vi "NicmosGlobal.vi"() -> ()   [LabVIEW 2009]
uses:
  Controls/NICMOS.MASKBANKS.ctl
  Controls/NICMOS.FILTERLIST.ctl
  Controls/NICMOS.FILTER.ctl
panel:
  out "BansMasksSquare":T1(array[cluster])
  in  "FilterList":T2
  in  "NI-DAQmx Task":refnum<k21>="NICMOS-DATA-TASK"
  in  "MASKBANKS":T4
  in  "Frame rate":dbl[unit]
  out "t__xx":i32=84
  out "txx__":i32=21
  out "Deglitch":i32=10
  out "Buffer Size":u32=1278
  out "Read Number":i32=138
  in  "Wheel Timeout":i32=90000
  in  "General Timeout":u32=10000
  out "Port Nicmos":refnum<visa-resource-name>="COM104"
  out "Reform Y":i32[](array[numeric])=[1, 1, 9, 9, 9, 9, 100]
  out "Reform X":i32[](array[numeric])=[1, 1, 9, 1, 9, 50, 100]
  out "Max Frequency":dbl[unit][](array[numeric])=[153846.15384615387, 105263.15789473684, 2442.002442002442, 3421.7279726261763, 2385.211687537269, 935.2349777881694, 48.14462645787947] format="%.2f"
  out "Min Frequency":dbl[unit][](array[numeric])=[238.2370458606313, 238.06689679800022, 217.36767742636667, 223.0524730942954, 216.90797679084645, 190.1050330307495, 40.061293779482604] format="%.2f"
  out "Bank Base Time":dbl[unit][](array[numeric])=[6.499999999999999e-06, 9.5e-06, 0.0004095, 0.00029225, 0.00041924999999999997, 0.0010692499999999999, 0.02077075] format="%.2f"
  out "Bank Size":i32[](array[numeric])=[1, 1, 81, 9, 81, 450, 10000]
  out "Current Bank":i32=3
  # "__________________  Timing  _________________"
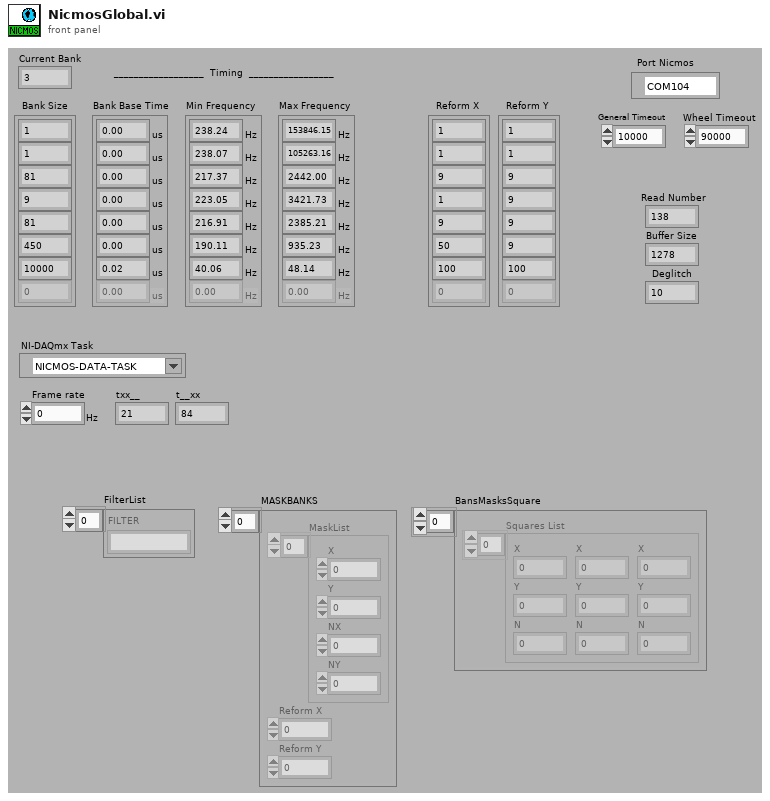
[diagram p1: front panel]
types:
  T1 = cluster{"Squares List":cluster{"X":i32, "Y":i32, "N":i32}[]}[]
  T2 = typedef "NICMOS.FILTERLIST.ctl" = T3[]
  T3 = typedef "NICMOS.FILTER.ctl" = string
  T4 = typedef "NICMOS.MASKBANKS.ctl" = cluster{"MaskList":cluster{"X":i32, "Y":i32, "NX":i32, "NY":i32}[], "Reform X":i32, "Reform Y":i32}[]
diagram:
